vi "switchboard_channel_mapping.vi"(3 "error in":errorcluster, 5 "Input parameters":T1={"Measurement type"=enum."Debug", "Sensor type"=enum."HPK_8in_256", "Identifier"="test.txt", "Open after execution?"=FALSE, "Plot after execution?"=FALSE, "Display channel"=0, "Voltage Delay (s)"=0.5, "Switch Delay (s)"=0.01, "VISA resource name source"="", "VISA resource name DMM"="", "VISA resource name LCR"="", "Compliance  Level (A)"=10.0, "Voltage Limit (V)"=1000.0, "Data storage location"="", "Scan voltages"="", "Use source as DMM?"=FALSE, "LCR signal frequenzy (Hz)"=10.0, "DMM device"=enum."Keithley2001", "Sampling number"=1, "Use env. sensors on"=enum."Sensirion sht1x/7x", "Switchboard Handle"=0, "Use Switchboard"=FALSE, "LCR signal voltage (V)"=10000.0, "Repeat"=1, "Scan voltages IV"="", "Scan voltages CV"="", "Hex pad numbers?"=FALSE, "Set measurement type"=enum."Debug", "Custom pad scan"="", "IV voltage Delay (s)"=0.5, "CV voltage Delay (s)"=0.5, "Needle measurement?"=FALSE, "Comments"="test.txt", "LCR signal frequenzy (kHz)"=10.0, "Compliance  Level (uA)"=10.0, "Open Correction Array"=array2304x3[6912 elements], "Current set voltage"=0.0, "Last set voltage"=0.0, "Current channel"=0, "Last OpenCorrection index"=-1, "Total curr/vltg every x steps"=10, "Current channel iteration"=0, "No CV corrections"=FALSE, "Mapfile"="", "Corrfile"="", "IV voltage file"=path "", "CV voltage file"=path "", "IV Switch Delay (s)"=0.01, "CV Switch Delay (s)"=0.01} {"CV Switch Delay (s)" format="%#_13g"; "IV Switch Delay (s)" format="%#_13g"; "Last set voltage" format="%#_13g"; "Current set voltage" format="%#_13g"; "CV voltage Delay (s)" format="%#_13g"; "IV voltage Delay (s)" format="%#_13g"; "Voltage Limit (V)" format="%#_13g"; "Voltage Delay (s)" format="%#_13g"; "Switch Delay (s)" format="%#_13g"}) -> (0 "error out":errorcluster, 1 "Custom pad array":i32[](array[numeric]), 2 "Channel array":i32[](array[numeric])=[255, 309, 187, 232, 316, 313, 383, 125, 177, 246, 235, 303, 372, 444, 445, 56, 112, 190, 189, 234, 318, 301, 375, 432, 508, 511, 58, 124, 127, 176, 254, 233, 311, 374, 442, 447, 498, 509, 60, 114, 188, 191, 236, 314, 317, 373, 434, 506, 503, 61, 126, 119, 178, 252, 245, 297, 382, 440, 439, 500, 507, 62, 113, 186, 185, 247, 298, 319, 371, 436, 504, 505, 59, 118, 123, 179, 250, 253, 306, 380, 377, 437, 502, 501, 57, 115, 182, 248, 249, 237, 299, 369, 438, 441, 499, 120, 116, 121, 181, 240, 251, 312, 378, 379, 435, 510, 497, 122, 117, 180, 238, 241, 308, 315, 368, 446, 443, 496, 184, 183, 242, 239, 302, 376, 381, 433, 244, 243, 304, 307, 370, 300, 305, 310, 296, 40, 41, 42, 43, 44, 45, 46, 47, 63, 48, 49, 50, 51, 52, 53, 54, 55])   [LabVIEW 2016]
doc: "Reads the switchboard to probe card map and set corresponding channel list."
uses:
  input_params.ctl
panel:
  out "subarray":string[][](array[string])
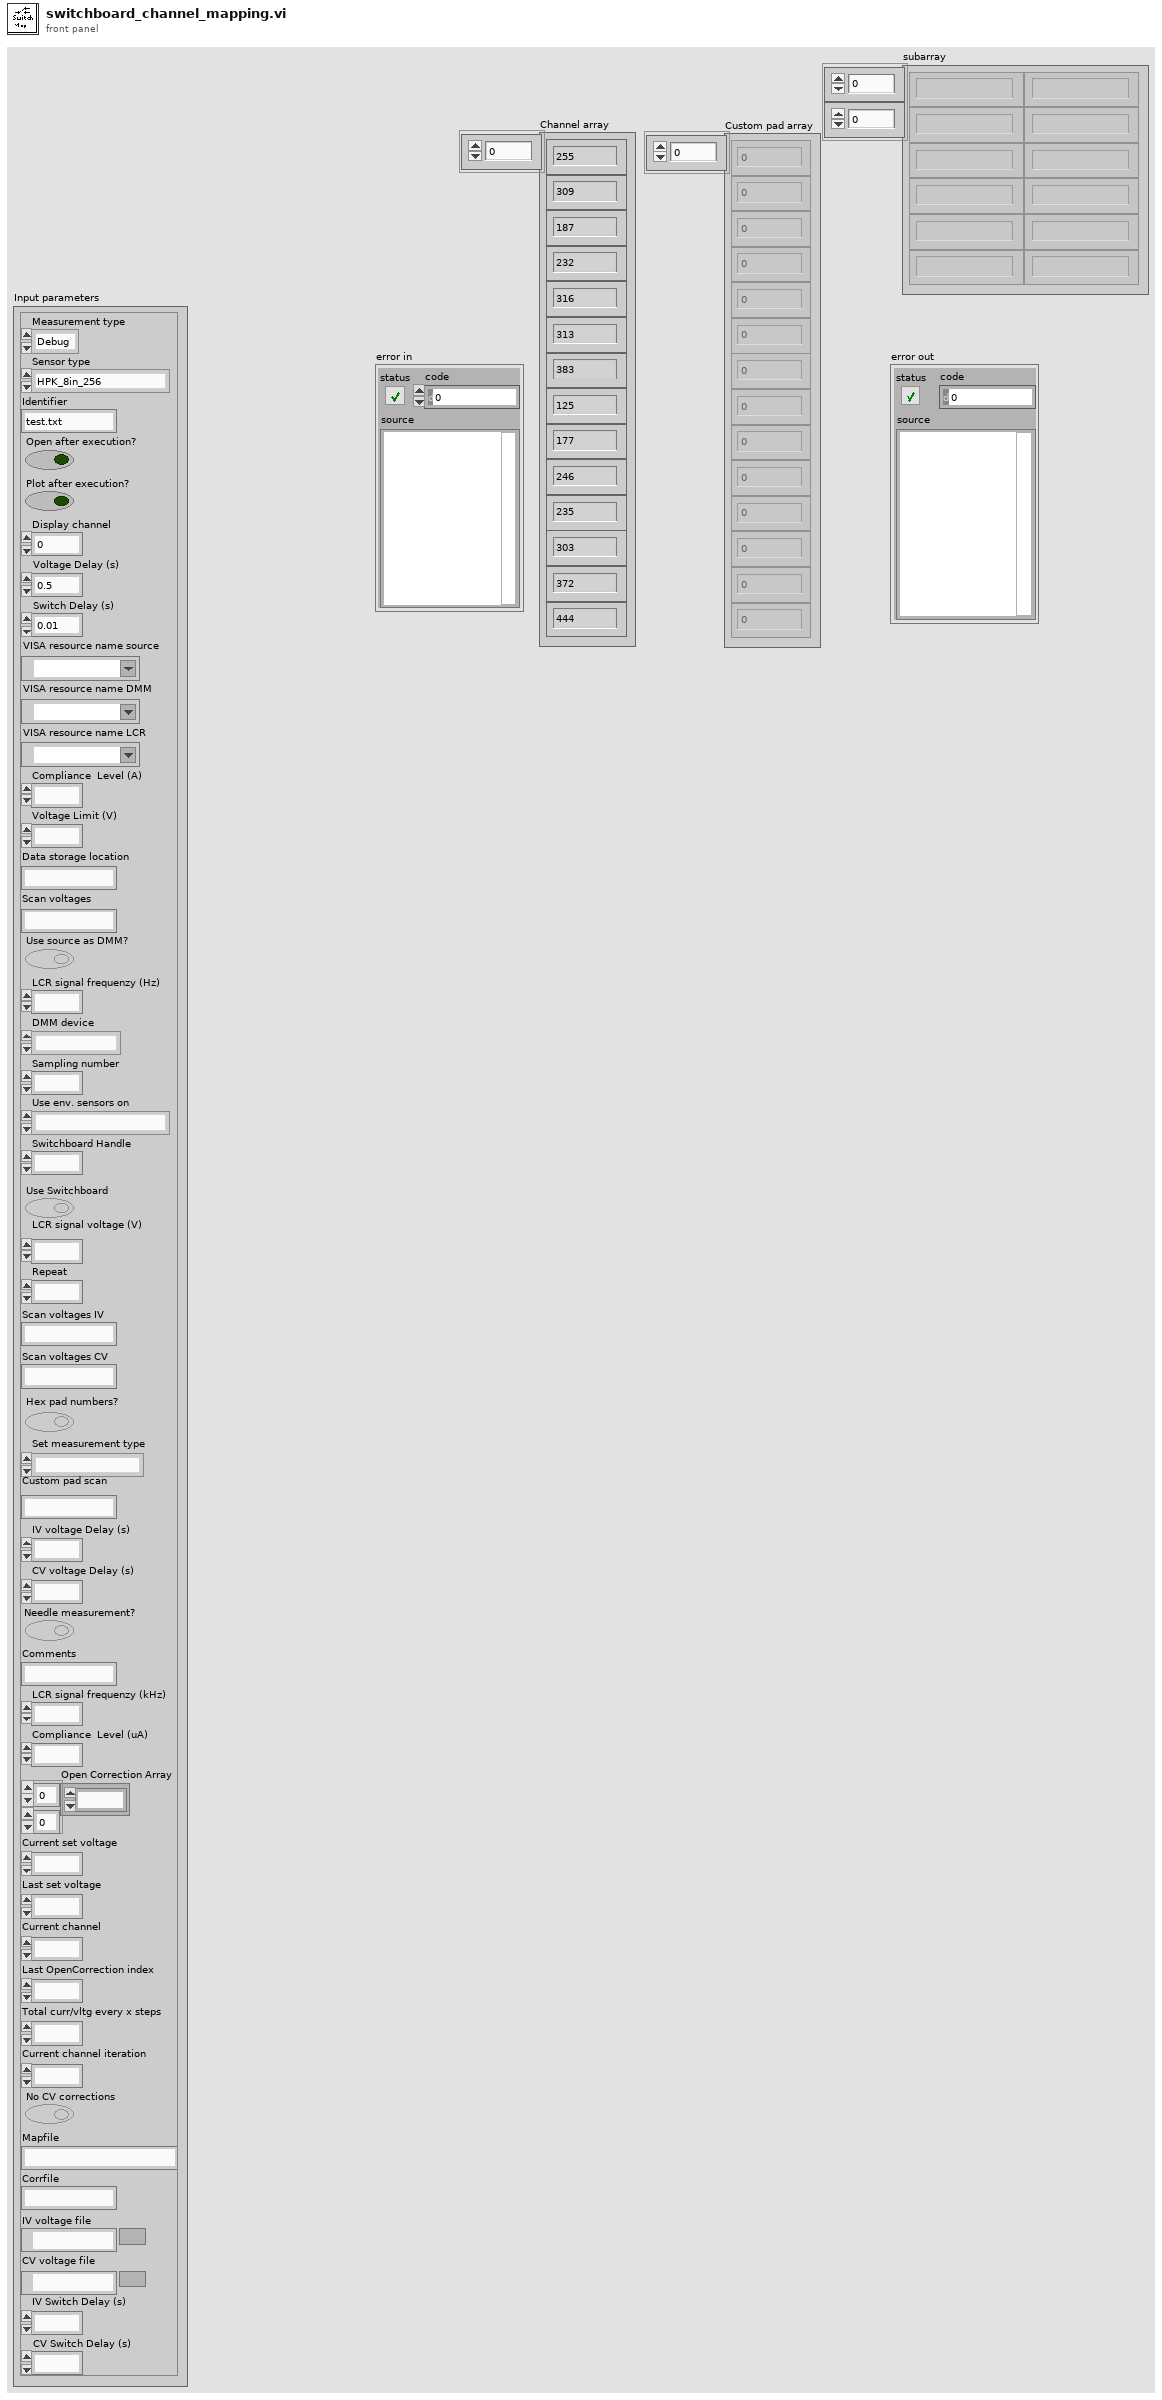
[diagram p1: front panel]
types:
  T1 = typedef "input_params.ctl" = cluster{"Measurement type":enum16{"IV", "CV", "Debug", "Test_contact"}, "Sensor type":enum16{"HPK_6in_135", "HPK_8in_256", "IFX_8in_256", "Diode", "HPK_6in_256", "Full matrix"}, "Identifier":string, "Open after execution?":bool, "Plot after execution?":bool, "Display channel":i32, "Voltage Delay (s)":dbl, "Switch Delay (s)":dbl, "VISA resource name source":refnum<visa-resource-name>, "VISA resource name DMM":refnum<visa-resource-name>, "VISA resource name LCR":refnum<visa-resource-name>, "Compliance  Level (A)":dbl, "Voltage Limit (V)":dbl, "Data storage location":string, "Scan voltages":string, "Use source as DMM?":bool, "LCR signal frequenzy (Hz)":dbl, "DMM device":enum16{"Keithley2001", "Keithley2450", "Keithley2410", "Keithley6487"}, "Sampling number":i32, "Use env. sensors on":enum16{"Sensirion sht1x/7x", "Switch Matrix", "Probecard"}, "Switchboard Handle":u32, "Use Switchboard":bool, "LCR signal voltage (V)":dbl, "Repeat":i32, "Scan voltages IV":string, "Scan voltages CV":string, "Hex pad numbers?":bool, "Set measurement type":enum16{"IV", "CV", "Debug", "Test_contact", "IV+CV"}, "Custom pad scan":string, "IV voltage Delay (s)":dbl, "CV voltage Delay (s)":dbl, "Needle measurement?":bool, "Comments":string, "LCR signal frequenzy (kHz)":dbl, "Compliance  Level (uA)":dbl, "Open Correction Array":dbl[][], "Current set voltage":dbl, "Last set voltage":dbl, "Current channel":i32, "Last OpenCorrection index":i32, "Total curr/vltg every x steps":i32, "Current channel iteration":i32, "No CV corrections":bool, "Mapfile":string, "Corrfile":string, "IV voltage file":path, "CV voltage file":path, "IV Switch Delay (s)":dbl, "CV Switch Delay (s)":dbl}
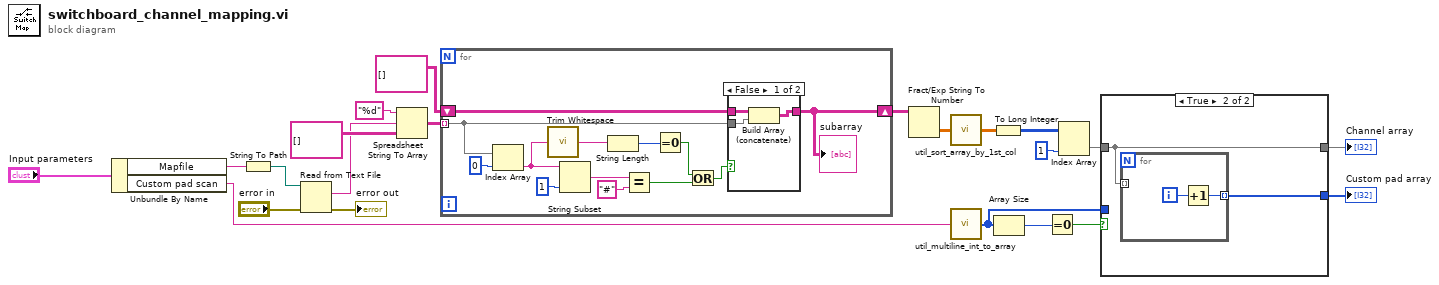
[diagram p0: block diagram]
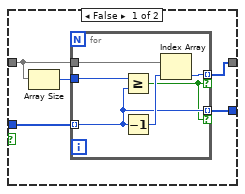
[diagram p3: hidden frame]
diagram:
  n1 = Unbundle By Name("Input parameters") -> ("Mapfile"=w14:string, "Custom pad scan"=w21:string)
  n2 = String To Path(string=w14) -> (path=w6:path)
  n3 = Read from Text File(file (use dialog)=w6, error in="error in") -> (text=w7:string, error out=→"error out":errorcluster)  [unwired: 2 in, 2 out]
  n4 = Spreadsheet String To Array(format string="%d", spreadsheet string=w7, array type (2D Dbl)=string[][] [] ("Array")) -> (array=w5:string[][])  [unwired: 1 in]
  n5 = for {
    shift-right: [w26] -> w11
    shift-left: string[][] [] ("subarray") -> [w27]
    tunnel: w5 -> [w24] mode=indexing
    n6 = Index Array(array=w24, index=0 ("index (row)")) -> (element=w25:string)
    n7 = call <vilib>:"Trim Whitespace.vi"("string"=w25) -> ("trimmed string"=w31:string)  [unwired: 1 in]
    n8 = String Subset(string=w25, length (rest)=1 ("length (rest)")) -> (substring=w34:string)  [unwired: 1 in]
    n9 = String Length(string=w31) -> (length=w32:i32)
    n10 = Equal?(x=w34, y="#") -> (x = y?=w29:bool)
    n11 = Equal To 0?(x=w32) -> (x = 0?=w30:bool)
    n12 = Or(x=w30, y=w29) -> (x .or. y?=w28:bool)
    n13 = case shown="False" w28 {
      tunnel: w27 -> [w38 w39]
      tunnel: [w37 w39] -> w26
      tunnel: w24 -> [w36 _]
      frame False {
        n14 = Build Array (concatenate)(w38, w36) -> (w37:string[][])
      }
      frame True {
      }
    }
    "subarray" <- w26
  }
  n15 = Fract/Exp String To Number(string=w11) -> (number=w4:dbl[][])  [unwired: 3 in, 1 out]
  n16 = call "util_sort_array_by_1st_col.vi"("2D array to sort"=w4) -> ("Sorted array"=w3:dbl[][])
  n17 = call "util_multiline_int_to_array.vi"("Multiline integer string"=w21) -> ("Array"=w17:i32[])
  n18 = To Long Integer(number=w3) -> (32bit integer=w2:i32[][])
  n19 = Array Size(array=w17) -> (size(s)=w16:i32)
  n20 = Equal To 0?(x=w16) -> (x = 0?=w15:bool)
  n21 = Index Array(array=w2, index (col)=1 ("disabled index (col)")) -> (element=w20:i32[])  [unwired: 1 in]
  n22 = case shown="True" w15 {
    tunnel: w17 -> [w43 _]
    tunnel: w20 -> [w41 w52]
    tunnel: [w44 w52] -> w19
    tunnel: [w42 w51] -> w18
    frame False {
      n23 = Array Size(array=w41) -> (size(s)=w40:i32)
      n24 = for {
        tunnel: w43 -> [w46] mode=indexing
        tunnel: w41 -> [w50]
        tunnel: [w49] -> w44 mode=indexing if=w45
        tunnel: [w46] -> w42 mode=indexing if=w45
        tunnel: w40 -> [w47]
        n25 = Greater Or Equal?(x=w47, y=w46) -> (x >= y?=w45:bool)
        n26 = Decrement(x=w46) -> (x-1=w48:i32)
        n27 = Index Array(array=w50, index=w48) -> (element=w49:i32)
      }
    }
    frame True {
      n28 = for {
        tunnel: w52 -> [_] mode=indexing
        tunnel: [w53] -> w51 mode=indexing
        i -> [w54]
        n29 = Increment(x=w54) -> (x+1=w53:i32)
      }
    }
  }
  "Channel array" <- w19
  "Custom pad array" <- w18
